vi "MCM Quartal Group.vi"(4 "Sampling Rate":dbl, 5 "Symbol Rate":i32=1, 6 "Starting Subcarrier":dbl, 7 "QAM Comparison":enum16{"MT Modulate", "Homebrew"}(ring), 8 "DataLen":i32=512, 9 "QAM Complexity":T3(ring), 10 "Carrier Method":T2(ring), 11 "Lowest f":dbl=1.0 format="%0.2p") -> (0 "FFT Complex":cluster{"f0":dbl, "df":dbl, "real part":dbl[]}(graph), 1 "FFT Real":cluster{"f0":dbl, "df":dbl, "real part":dbl[]}(graph), 2 "output waveform":waveform(cdb), 3 "Waveform Chart":dbl[][](graph))   [LabVIEW 2018]
uses:
  <vilib>/Analysis/Matrix/Datatypes/ComplexMatrix.ctl
  <vilib>/measure/maspectr.llb/FFT Spectrum (Real-Im) for 1 Chan.vi
  <vilib>/measure/NI_MAPro.lvlib
  <vilib>/Analysis/Matrix/NI_Matrix.lvlib
  <vilib>/addons/Modulation/niDMT.lvlib
panel:
  out "Constellation Graph":T1(graph)
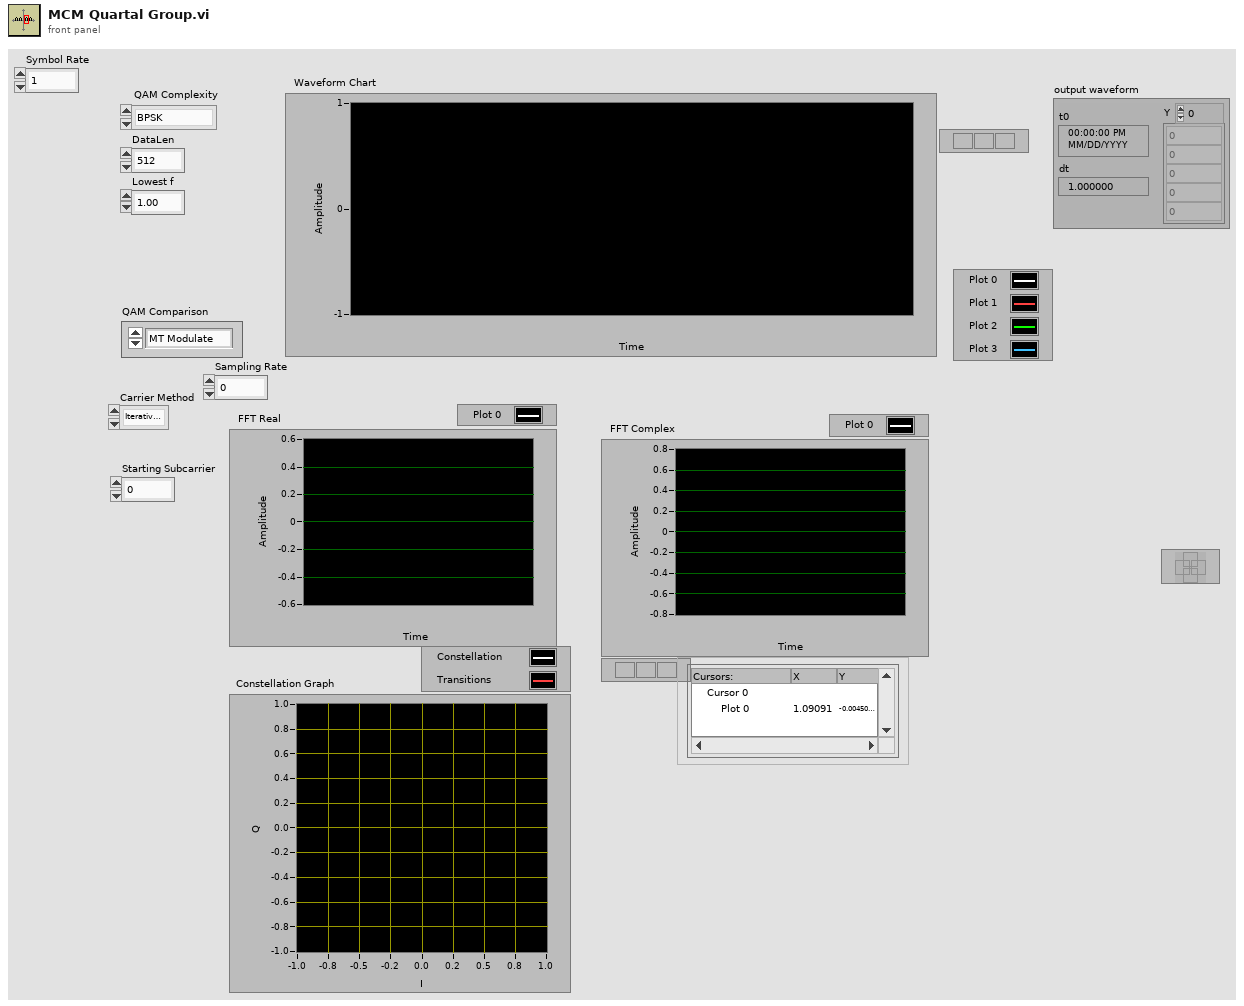
[diagram p1: front panel]
types:
  T1 = cluster{"Decimated Array":dbl[], "Decimated Array":dbl[]}[]
  T2 = enum16{"Iterative (Non-Reentrant)", "Crafted (Reentrant)"}
  T3 = enum16{"BPSK", "QPSK", "16-QAM", "64-QAM", "256-QAM"}
  T4 = typedef "NI_Matrix.lvlib/ComplexMatrix.ctl" = cdb[][]
  T5 = cluster{"f0":dbl, "df":dbl, "imaginary part":dbl[]}
  T6 = cluster{"constellation":dbl[], "oversampled data":dbl[]}[]
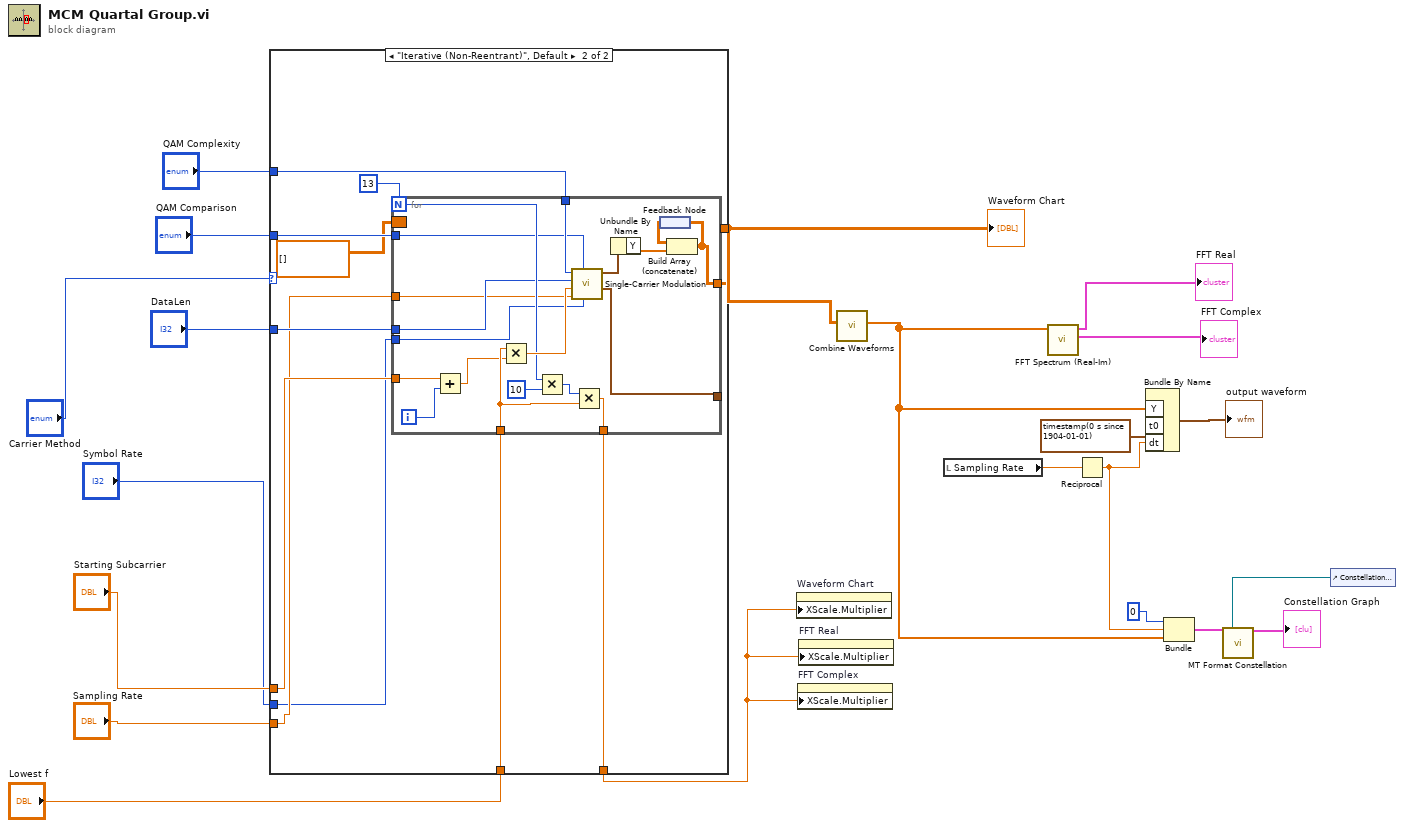
[diagram p0: block diagram]
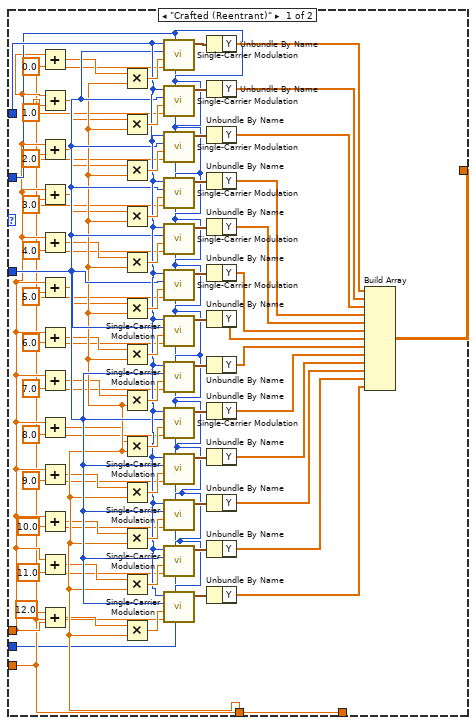
[diagram p2: hidden frame]
diagram:
  n1 = case shown="\"Iterative (Non-Reentrant)\", Default" "Carrier Method" {
    tunnel: "Lowest f" -> [w52 w105]
    tunnel: "DataLen" -> [w55 w104]
    tunnel: "QAM Complexity" -> [w56 w103]
    tunnel: "QAM Comparison" -> [w54 w102]
    tunnel: [w53 w100] -> w5
    tunnel: [w23 w99] -> w14
    tunnel: "Starting Subcarrier" -> [w37 w97]
    tunnel: "Sampling Rate" -> [w23 w96]
    tunnel: "Symbol Rate" -> [w22 w95]
    frame "Crafted (Reentrant)" {
      n2 = Add(x=w37, y=0.0 ("x")) -> (x+y=w25:dbl)
      n3 = Add(x=w37, y=1.0 ("x")) -> (x+y=w26:dbl)
      n4 = Add(x=w37, y=2.0 ("x")) -> (x+y=w27:dbl)
      n5 = Add(x=w37, y=3.0 ("x")) -> (x+y=w28:dbl)
      n6 = Add(x=w37, y=4.0 ("x")) -> (x+y=w29:dbl)
      n7 = Add(x=w37, y=5.0 ("x")) -> (x+y=w30:dbl)
      n8 = Add(x=w37, y=6.0 ("x")) -> (x+y=w31:dbl)
      n9 = Add(x=w37, y=7.0 ("x")) -> (x+y=w32:dbl)
      n10 = Add(x=w37, y=8.0 ("x")) -> (x+y=w33:dbl)
      n11 = Add(x=w37, y=9.0 ("x")) -> (x+y=w34:dbl)
      n12 = Add(x=w37, y=10.0 ("x")) -> (x+y=w35:dbl)
      n13 = Add(x=w37, y=11.0 ("x")) -> (x+y=w36:dbl)
      n14 = Add(x=12.0, y=w37) -> (x+y=w50:dbl)
      n15 = Multiply(x=w25, y=w52) -> (x*y=w57:dbl)
      n16 = Multiply(x=w26, y=w52) -> (x*y=w60:dbl)
      n17 = Multiply(x=w27, y=w52) -> (x*y=w61:dbl)
      n18 = Multiply(x=w28, y=w52) -> (x*y=w64:dbl)
      n19 = Multiply(x=w29, y=w52) -> (x*y=w65:dbl)
      n20 = Multiply(x=w30, y=w52) -> (x*y=w68:dbl)
      n21 = Multiply(x=w31, y=w52) -> (x*y=w80:dbl)
      n22 = Multiply(x=w32, y=w52) -> (x*y=w77:dbl)
      n23 = Multiply(x=w33, y=w52) -> (x*y=w76:dbl)
      n24 = Multiply(x=w34, y=w52) -> (x*y=w73:dbl)
      n25 = Multiply(x=w35, y=w52) -> (x*y=w72:dbl)
      n26 = Multiply(x=w36, y=w52) -> (x*y=w69:dbl)
      n27 = Multiply(x=w50, y=w52) -> (x*y=w24:dbl)
      n28 = call "Single-Carrier Modulation.vi"("Symbol Rate"=w22, "QAM Comparison"=w54, "Sampling Rate"=w23, "frequency"=w57, "DataLen"=w55, "QAM Complexity"=w56) -> ("waveform"=w58:waveform(cdb))  [unwired: 4 in, 1 out]
      n29 = call "Single-Carrier Modulation.vi"("Symbol Rate"=w22, "QAM Comparison"=w54, "Sampling Rate"=w23, "frequency"=w60, "DataLen"=w55, "QAM Complexity"=w56) -> ("waveform"=w59:waveform(cdb))  [unwired: 4 in, 1 out]
      n30 = call "Single-Carrier Modulation.vi"("Symbol Rate"=w22, "QAM Comparison"=w54, "Sampling Rate"=w23, "frequency"=w61, "DataLen"=w55, "QAM Complexity"=w56) -> ("waveform"=w62:waveform(cdb))  [unwired: 4 in, 1 out]
      n31 = call "Single-Carrier Modulation.vi"("Symbol Rate"=w22, "QAM Comparison"=w54, "Sampling Rate"=w23, "frequency"=w64, "DataLen"=w55, "QAM Complexity"=w56) -> ("waveform"=w63:waveform(cdb))  [unwired: 4 in, 1 out]
      n32 = call "Single-Carrier Modulation.vi"("Symbol Rate"=w22, "QAM Comparison"=w54, "Sampling Rate"=w23, "frequency"=w65, "DataLen"=w55, "QAM Complexity"=w56) -> ("waveform"=w66:waveform(cdb))  [unwired: 4 in, 1 out]
      n33 = call "Single-Carrier Modulation.vi"("Symbol Rate"=w22, "QAM Comparison"=w54, "Sampling Rate"=w23, "frequency"=w68, "DataLen"=w55, "QAM Complexity"=w56) -> ("waveform"=w67:waveform(cdb))  [unwired: 4 in, 1 out]
      n34 = call "Single-Carrier Modulation.vi"("Symbol Rate"=w22, "QAM Comparison"=w54, "Sampling Rate"=w23, "frequency"=w80, "DataLen"=w55, "QAM Complexity"=w56) -> ("waveform"=w79:waveform(cdb))  [unwired: 4 in, 1 out]
      n35 = call "Single-Carrier Modulation.vi"("Symbol Rate"=w22, "QAM Comparison"=w54, "Sampling Rate"=w23, "frequency"=w77, "DataLen"=w55, "QAM Complexity"=w56) -> ("waveform"=w78:waveform(cdb))  [unwired: 4 in, 1 out]
      n36 = call "Single-Carrier Modulation.vi"("Symbol Rate"=w22, "QAM Comparison"=w54, "Sampling Rate"=w23, "frequency"=w76, "DataLen"=w55, "QAM Complexity"=w56) -> ("waveform"=w75:waveform(cdb))  [unwired: 4 in, 1 out]
      n37 = call "Single-Carrier Modulation.vi"("Symbol Rate"=w22, "QAM Comparison"=w54, "Sampling Rate"=w23, "frequency"=w73, "DataLen"=w55, "QAM Complexity"=w56) -> ("waveform"=w74:waveform(cdb))  [unwired: 4 in, 1 out]
      n38 = call "Single-Carrier Modulation.vi"("Symbol Rate"=w22, "QAM Comparison"=w54, "Sampling Rate"=w23, "frequency"=w72, "DataLen"=w55, "QAM Complexity"=w56) -> ("waveform"=w71:waveform(cdb))  [unwired: 4 in, 1 out]
      n39 = call "Single-Carrier Modulation.vi"("Symbol Rate"=w22, "QAM Comparison"=w54, "Sampling Rate"=w23, "frequency"=w69, "DataLen"=w55, "QAM Complexity"=w56) -> ("waveform"=w70:waveform(cdb))  [unwired: 4 in, 1 out]
      n40 = call "Single-Carrier Modulation.vi"("Symbol Rate"=w22, "QAM Comparison"=w54, "Sampling Rate"=w23, "frequency"=w24, "DataLen"=w55, "QAM Complexity"=w56) -> ("waveform"=w81:waveform(cdb))  [unwired: 4 in, 1 out]
      n41 = Unbundle By Name(w58) -> ("Y"=w82:cdb[])
      n42 = Unbundle By Name(w59) -> ("Y"=w83:cdb[])
      n43 = Unbundle By Name(w62) -> ("Y"=w84:cdb[])
      n44 = Unbundle By Name(w63) -> ("Y"=w85:cdb[])
      n45 = Unbundle By Name(w66) -> ("Y"=w86:cdb[])
      n46 = Unbundle By Name(w67) -> ("Y"=w87:cdb[])
      n47 = Unbundle By Name(w79) -> ("Y"=w88:cdb[])
      n48 = Unbundle By Name(w78) -> ("Y"=w89:cdb[])
      n49 = Unbundle By Name(w75) -> ("Y"=w90:cdb[])
      n50 = Unbundle By Name(w74) -> ("Y"=w91:cdb[])
      n51 = Unbundle By Name(w71) -> ("Y"=w92:cdb[])
      n52 = Unbundle By Name(w70) -> ("Y"=w93:cdb[])
      n53 = Unbundle By Name(w81) -> ("Y"=w94:cdb[])
      n54 = Build Array(w82, w83, w84, w85, w86, w87, w88, w89, w90, w91, w92, w93, w94) -> (w53:T4)
    }
    frame "Iterative (Non-Reentrant)", Default {
      n55 = for {
        N: 13 -> [w123]
        tunnel: w105 -> [w116]
        tunnel: w104 -> [w121]
        tunnel: w103 -> [w120]
        tunnel: w102 -> [w119]
        tunnel: [w118] -> _
        tunnel: [w112] -> w100
        border: T4 [] ("Complex Matrix") -> [_]
        tunnel: [w111] -> w99
        tunnel: w97 -> [w108]
        tunnel: w96 -> [w107]
        tunnel: w95 -> [w106]
        i -> [w110]
        n56 = Add(x=w108, y=w110) -> (x+y=w109:dbl)
        n57 = Multiply(x=w116, y=w109) -> (x*y=w124:dbl)
        n58 = Multiply(x=w123, y=10) -> (x*y=w117:i32)
        n59 = call "Single-Carrier Modulation.vi"("Symbol Rate"=w106, "QAM Comparison"=w119, "Sampling Rate"=w107, "frequency"=w124, "DataLen"=w121, "QAM Complexity"=w120) -> ("sampling info"=w118:cluster{"Fs":dbl, "#s":dbl}, "waveform"=w115:waveform(cdb))  [unwired: 4 in]
        n60 = Multiply(x=w117, y=w116) -> (x*y=w111:dbl)
        n61 = Unbundle By Name(w115) -> ("Y"=w114:cdb[])
        n62 = feedback #1() -> (w113:T4)
        n63 = Build Array (concatenate)(w113, w114) -> (w112:T4)
        n64 = feedback-in #1(w112) -> ()
      }
    }
  }
  "Waveform Chart" <- w5
  n65 = property on="Waveform Chart" class="WFChart (strict)"("XScale.Multiplier"=w14) -> ()  [unwired: 2 in, 2 out]
  n66 = property on="FFT Complex" class="WFGraph (strict)"("XScale.Multiplier"=w14) -> ()  [unwired: 2 in, 2 out]
  n67 = property on="FFT Real" class="WFGraph (strict)"("XScale.Multiplier"=w14) -> ()  [unwired: 2 in, 2 out]
  n68 = call "Combine Waveforms.vi"("Matrix of Carriers"=w5) -> ("Combined Output"=w6:cdb[])  [unwired: 10 in]
  n69 = local read "Sampling Rate"() -> (w2:dbl)
  n70 = call-poly <vilib>:"FFT Spectrum (Real-Im).vi"("time signal"=w6) -> ("imaginary part"=→"FFT Complex":T5, "real part"=→"FFT Real":cluster{"f0":dbl, "df":dbl, "real part":dbl[]})  [unwired: 6 in, 3 out]
  n71 = Reciprocal(x=w2) -> (1/x=w7:dbl)
  n72 = Bundle By Name("Y"=w6, "t0"=timestamp(0 s since 1904-01-01), "dt"=w7) -> (→"output waveform":waveform(cdb))  [unwired: 1 in]
  n73 = Bundle(0, w7, "Combined Output"=w6) -> (w9:cluster{i32, dbl, "Combined Output":cdb[]})  [unwired: 1 in]
  n74 = control-ref of="Constellation Graph"() -> (w12:refnum<vi>)
  n75 = call <vilib>:"MT Format Constellation.vi"("waveform"=w9, "constellation reference"=w12) -> ("constellation graph"=→"Constellation Graph":T6)  [unwired: 3 in, 10 out]
